vi "BBoxLite28A.vi"() -> ()   [LabVIEW 2020]
uses:
  Y:/Documents/TMYtek/Code/bbox-api/example/BBoxLite Series/BBoxLite 5G/LabVIEW/BBoxLite28A/BBoxAPI.dll
  BBoxAPI.dll
panel:
  out "getAAKitList":string[](array[string])
  out "setBeamAngle":i32
  in  "Phi":i32 min=-45 max=45 step=1
  out "switchChannelPower":string
  in  "Power":i32
  out "selectAAKit":i32(ring) items=["OK"=0, "WARNING"=1, "ERROR"=2, "NO_RESPONSE"=3, "ERROR_GET_SN"=10, "ERROR_DEV_TYPE"=11, "ERROR_INIT_OBJECT"=12, "ERROR_DEV_NOT_INIT"=13, "ERROR_METHOD_NOT_FOUND"=14, "ERROR_REFLECTION"=15, "ERROR_POWER"=16, "ERROR_NETWORK_NOT_INIT"=20, "ERROR_NETWORK_INIT"=21, "ERROR_NETWORK_CONNECT_TIMEOUT"=22, "ERROR_DISCONNECT"=23, "ERROR_SOCKET"=24, "ERROR_SEND_CMD"=25, "ERROR_RESP_CMD"=26, "ERROR_DEV_COUNT_ZERO"=30, "ERROR_CMD"=40, "ERROR_CMD_INIT"=41, "ERROR_BF_AAKIT"=100, "ERROR_BF_NO_AAKIT"=101, "ERROR_BF_CALI_PATH"=102, "ERROR_BF_BEAMXY"=103, "ERROR_BF_GEN"=104, "ERROR_BF_TRMODE"=105, "STATUS_BF_LOAD_CALI_INCOMPLTE"=106, "ERROR_BF_LOAD_CALI_PARSE_FAILED"=107, "ERROR_FREQ_EQUATION"=250, "ERROR_PLO_CRC"=251, "WARNING_HARMONIC"=252, "ERROR_HARMONIC_BLOCK"=253]
  out "readBeamPhaseValues":i32[][](array[numeric])
  out "readBeamGainValues":dbl[][](array[numeric])
  in  "Theta":i32 min=-45 max=45 step=1
  in  "Beam Gain":dbl step=0.5
  out "setChannelGainPhase":string
  in  "Phase":i32 min=0 max=355 step=5
  in  "Gain":dbl=18.0 step=0.5
  in  "Channel":i32=1 min=1 max=4
  in  "TxRxMode":i32=1 min=1 max=2 step=1
  out "Maxmum Gain":dbl
  out "Minimum Gain":dbl
  out "getTxRxMode":i32
  out "SwitchTxRxMode":i32(ring) items=["OK"=0, "WARNING"=1, "ERROR"=2, "NO_RESPONSE"=3, "ERROR_GET_SN"=10, "ERROR_DEV_TYPE"=11, "ERROR_INIT_OBJECT"=12, "ERROR_DEV_NOT_INIT"=13, "ERROR_METHOD_NOT_FOUND"=14, "ERROR_REFLECTION"=15, "ERROR_POWER"=16, "ERROR_NETWORK_NOT_INIT"=20, "ERROR_NETWORK_INIT"=21, "ERROR_NETWORK_CONNECT_TIMEOUT"=22, "ERROR_DISCONNECT"=23, "ERROR_SOCKET"=24, "ERROR_SEND_CMD"=25, "ERROR_RESP_CMD"=26, "ERROR_DEV_COUNT_ZERO"=30, "ERROR_CMD"=40, "ERROR_CMD_INIT"=41, "ERROR_BF_AAKIT"=100, "ERROR_BF_NO_AAKIT"=101, "ERROR_BF_CALI_PATH"=102, "ERROR_BF_BEAMXY"=103, "ERROR_BF_GEN"=104, "ERROR_BF_TRMODE"=105, "STATUS_BF_LOAD_CALI_INCOMPLTE"=106, "ERROR_BF_LOAD_CALI_PARSE_FAILED"=107, "ERROR_FREQ_EQUATION"=250, "ERROR_PLO_CRC"=251, "WARNING_HARMONIC"=252, "ERROR_HARMONIC_BLOCK"=253]
  out "setOperatingFreq":i32(ring) items=["OK"=0, "WARNING"=1, "ERROR"=2, "NO_RESPONSE"=3, "ERROR_GET_SN"=10, "ERROR_DEV_TYPE"=11, "ERROR_INIT_OBJECT"=12, "ERROR_DEV_NOT_INIT"=13, "ERROR_METHOD_NOT_FOUND"=14, "ERROR_REFLECTION"=15, "ERROR_POWER"=16, "ERROR_NETWORK_NOT_INIT"=20, "ERROR_NETWORK_INIT"=21, "ERROR_NETWORK_CONNECT_TIMEOUT"=22, "ERROR_DISCONNECT"=23, "ERROR_SOCKET"=24, "ERROR_SEND_CMD"=25, "ERROR_RESP_CMD"=26, "ERROR_DEV_COUNT_ZERO"=30, "ERROR_CMD"=40, "ERROR_CMD_INIT"=41, "ERROR_BF_AAKIT"=100, "ERROR_BF_NO_AAKIT"=101, "ERROR_BF_CALI_PATH"=102, "ERROR_BF_BEAMXY"=103, "ERROR_BF_GEN"=104, "ERROR_BF_TRMODE"=105, "STATUS_BF_LOAD_CALI_INCOMPLTE"=106, "ERROR_BF_LOAD_CALI_PARSE_FAILED"=107, "ERROR_FREQ_EQUATION"=250, "ERROR_PLO_CRC"=251, "WARNING_HARMONIC"=252, "ERROR_HARMONIC_BLOCK"=253]
  out "getFrequencyList":string[](array[string])
  out "Init":i32(ring) items=["OK"=0, "WARNING"=1, "ERROR"=2, "NO_RESPONSE"=3, "ERROR_GET_SN"=10, "ERROR_DEV_TYPE"=11, "ERROR_INIT_OBJECT"=12, "ERROR_DEV_NOT_INIT"=13, "ERROR_METHOD_NOT_FOUND"=14, "ERROR_REFLECTION"=15, "ERROR_POWER"=16, "ERROR_NETWORK_NOT_INIT"=20, "ERROR_NETWORK_INIT"=21, "ERROR_NETWORK_CONNECT_TIMEOUT"=22, "ERROR_DISCONNECT"=23, "ERROR_SOCKET"=24, "ERROR_SEND_CMD"=25, "ERROR_RESP_CMD"=26, "ERROR_DEV_COUNT_ZERO"=30, "ERROR_CMD"=40, "ERROR_CMD_INIT"=41, "ERROR_BF_AAKIT"=100, "ERROR_BF_NO_AAKIT"=101, "ERROR_BF_CALI_PATH"=102, "ERROR_BF_BEAMXY"=103, "ERROR_BF_GEN"=104, "ERROR_BF_TRMODE"=105, "STATUS_BF_LOAD_CALI_INCOMPLTE"=106, "ERROR_BF_LOAD_CALI_PARSE_FAILED"=107, "ERROR_FREQ_EQUATION"=250, "ERROR_PLO_CRC"=251, "WARNING_HARMONIC"=252, "ERROR_HARMONIC_BLOCK"=253]
  out "SN":string
  out "ScanningDevice":string[](array[string])
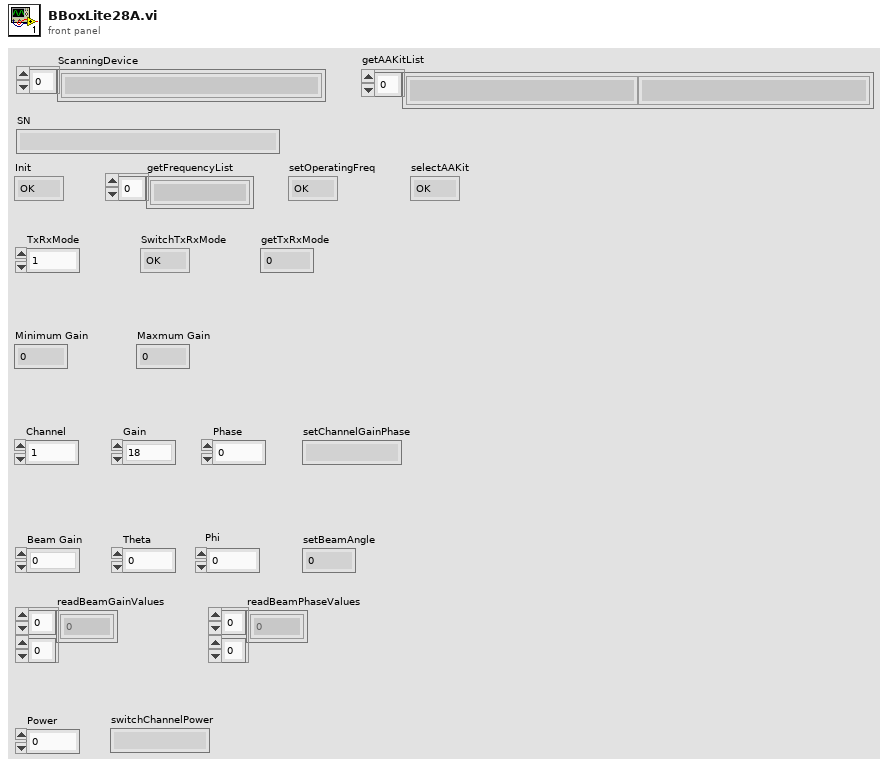
[diagram p1: front panel]
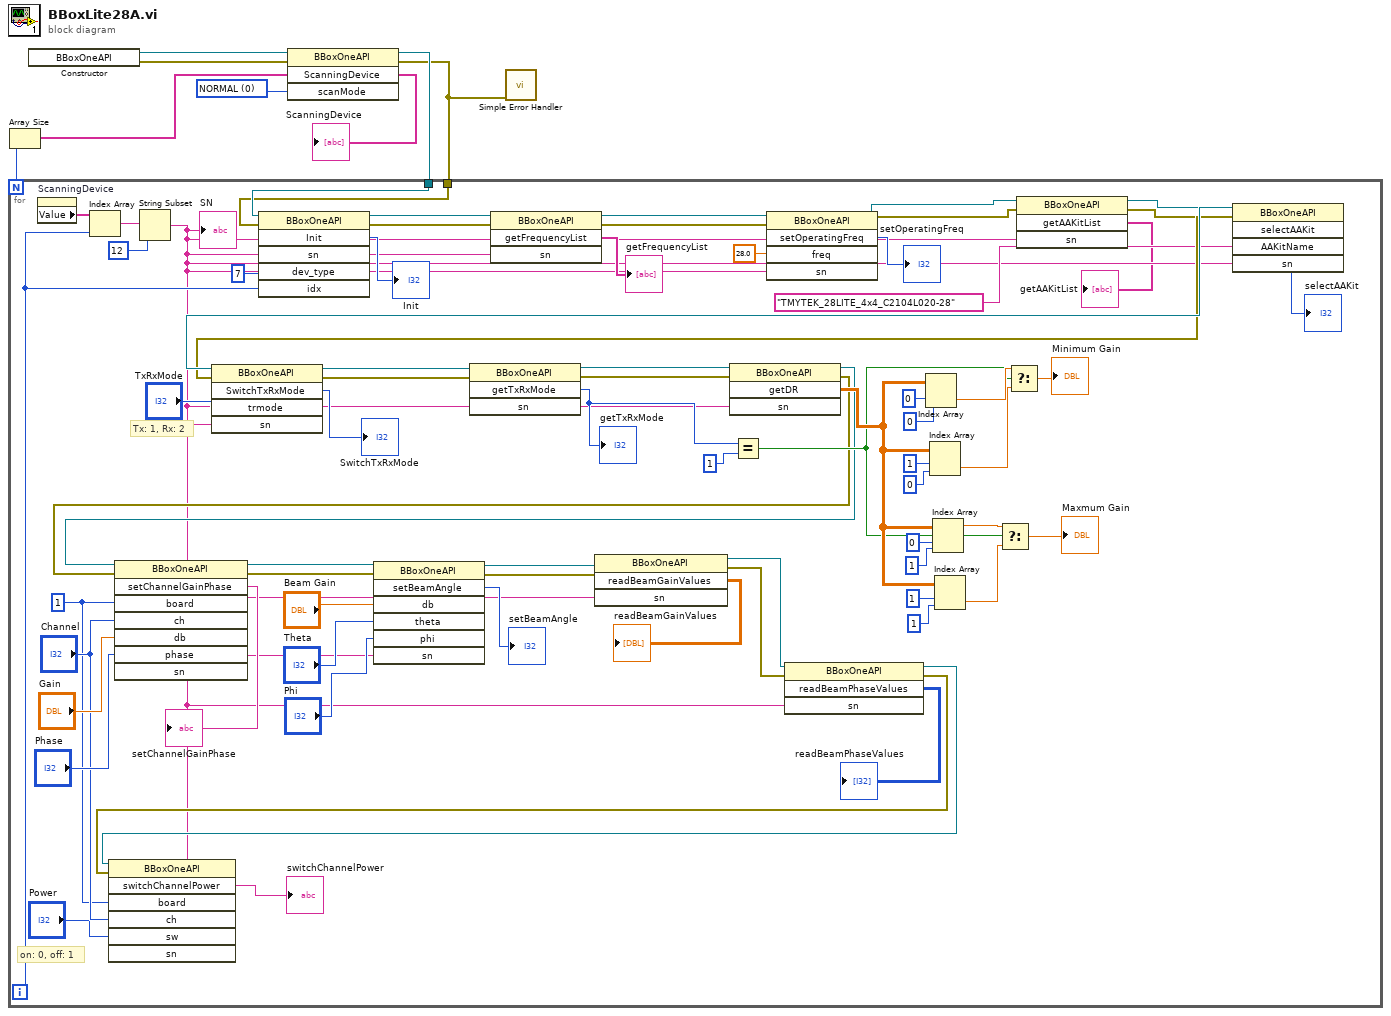
[diagram p0: block diagram]
diagram:
  w7 = 0 items=["NORMAL", "FAST"] ("scanMode")
  n1 = constructor class="BBoxOneAPI"() -> (reference out=w6:refnum<k24>, error out=w5:errorcluster)  [unwired: 3 in, 1 out]
  n2 = invoke class="BBoxOneAPI" method="ScanningDevice"(reference=w6, error in=w5, "scanMode"=w7) -> (reference out=w2:refnum<k24>, error out=w1:errorcluster, "ScanningDevice"=w3:string[])  [unwired: 1 in, 1 out]
  "ScanningDevice" <- w3
  n3 = Array Size(array=w3) -> (size(s)=w4:i32)
  n4 = for {
    N: w4 -> [_]
    tunnel: w2 -> [w77]
    tunnel: w1 -> [w76]
    i -> [w74]
    w19 = 1
    # "on: 0, off: 1"
    # "Tx: 1, Rx: 2"
    n5 = property on="ScanningDevice" class="Arr (strict)"() -> ("Value"=w8:string[])  [unwired: 2 in, 2 out]
    n6 = Index Array(array=w8, index=w74) -> (element=w79:string)
    n7 = String Subset(string=w79, length (rest)=12) -> (substring=w10:string)  [unwired: 1 in]
    "SN" <- w10
    n8 = invoke class="BBoxOneAPI" method="Init"(reference=w77, error in=w76, "sn"=w10, "dev_type"=7, "idx"=w74) -> (reference out=w72:refnum<k24>, error out=w71:errorcluster, "Init"=→"Init":i32)  [unwired: 1 in, 3 out]
    n9 = invoke on="Invoke Node" class="BBoxOneAPI" method="getFrequencyList"(reference=w72, error in=w71, "sn"=w10) -> (reference out=w69:refnum<k24>, error out=w68:errorcluster, "getFrequencyList"=→"getFrequencyList":string[])  [unwired: 1 in, 1 out]
    n10 = invoke class="BBoxOneAPI" method="setOperatingFreq"(reference=w69, error in=w68, "freq"=28.0, "sn"=w10) -> (reference out=w14:refnum<k24>, error out=w13:errorcluster, "setOperatingFreq"=→"setOperatingFreq":i32)  [unwired: 1 in, 2 out]
    n11 = invoke class="BBoxOneAPI" method="getAAKitList"(reference=w14, error in=w13, "sn"=w10) -> (reference out=w12:refnum<k24>, error out=w11:errorcluster, "getAAKitList"=→"getAAKitList":string[])  [unwired: 1 in, 1 out]
    n12 = invoke class="BBoxOneAPI" method="selectAAKit"(reference=w12, error in=w11, "AAKitName"="TMYTEK_28LITE_4x4_C2104L020-28", "sn"=w10) -> (reference out=w26:refnum<k24>, error out=w25:errorcluster, "selectAAKit"=→"selectAAKit":i32)  [unwired: 1 in, 2 out]
    n13 = invoke class="BBoxOneAPI" method="SwitchTxRxMode"(reference=w26, error in=w25, "trmode"="TxRxMode", "sn"=w10) -> (reference out=w64:refnum<k24>, error out=w63:errorcluster, "SwitchTxRxMode"=→"SwitchTxRxMode":i32)  [unwired: 1 in, 2 out]
    n14 = invoke class="BBoxOneAPI" method="getTxRxMode"(reference=w64, error in=w63, "sn"=w10) -> (reference out=w62:refnum<k24>, error out=w61:errorcluster, "getTxRxMode"=w60:i32)  [unwired: 1 in, 1 out]
    "getTxRxMode" <- w60
    n15 = invoke class="BBoxOneAPI" method="getDR"(reference=w62, error in=w61, "sn"=w10) -> (reference out=w41:refnum<k24>, error out=w40:errorcluster, "getDR"=w49:dbl[][])  [unwired: 1 in, 1 out]
    n16 = invoke class="BBoxOneAPI" method="setChannelGainPhase"(reference=w41, error in=w40, "board"=w19, "ch"="Channel", "db"="Gain", "phase"="Phase", "sn"=w10) -> (reference out=w36:refnum<k24>, error out=w35:errorcluster, "setChannelGainPhase"=→"setChannelGainPhase":string)  [unwired: 1 in, 5 out]
    n17 = invoke class="BBoxOneAPI" method="setBeamAngle"(reference=w36, error in=w35, "db"="Beam Gain", "theta"="Theta", "phi"="Phi", "sn"=w10) -> (reference out=w32:refnum<k24>, error out=w31:errorcluster, "setBeamAngle"=→"setBeamAngle":i32)  [unwired: 1 in, 4 out]
    n18 = invoke class="BBoxOneAPI" method="readBeamGainValues"(reference=w32, error in=w31, "sn"=w10) -> (reference out=w29:refnum<k24>, error out=w28:errorcluster, "readBeamGainValues"=→"readBeamGainValues":dbl[][])  [unwired: 1 in, 1 out]
    n19 = Equal?(x=w60, y=1) -> (x = y?=w46:bool)
    n20 = invoke class="BBoxOneAPI" method="readBeamPhaseValues"(reference=w29, error in=w28, "sn"=w10) -> (reference out=w22:refnum<k24>, error out=w21:errorcluster, "readBeamPhaseValues"=→"readBeamPhaseValues":i32[][])  [unwired: 1 in, 1 out]
    n21 = invoke class="BBoxOneAPI" method="switchChannelPower"(reference=w22, error in=w21, "board"=w19, "ch"="Channel", "sw"="Power", "sn"=w10) -> ("switchChannelPower"=→"switchChannelPower":string)  [unwired: 1 in, 6 out]
    n22 = Index Array(array=w49, index (row)=0, index (col)=0) -> (element=w56:dbl)
    n23 = Index Array(array=w49, index (row)=1, index (col)=0) -> (element=w53:dbl)
    n24 = Index Array(array=w49, index (row)=0, index (col)=1) -> (element=w45:dbl)
    n25 = Index Array(array=w49, index (row)=1, index (col)=1) -> (element=w44:dbl)
    n26 = Select(t=w45, s=w46, f=w44) -> (s? t:f=→"Maxmum Gain":dbl)
    n27 = Select(t=w56, s=w46, f=w53) -> (s? t:f=→"Minimum Gain":dbl)
  }
  n28 = call <vilib>:"Simple Error Handler.vi"("error in (no error)"=w1) -> ()  [unwired: 4 in, 5 out]
